vi "init.vi"(8 "error in (no error)":errorcluster, 11 "Relays in":refnum<class "Relays.lvclass">) -> (0 "error out":errorcluster, 3 "Relays out":refnum<class "Relays.lvclass">)   [LabVIEW 2025, in "Relays.lvclass"]
uses:
  Relays.lvclass
  Relays.lvclass/Relays.ctl
  Processor/Processor.lvclass
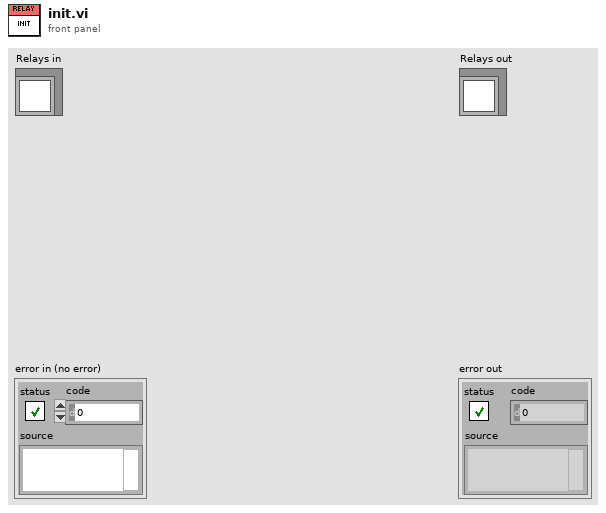
[diagram p1: front panel]
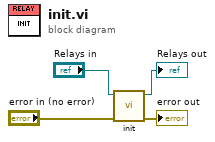
[diagram p0: block diagram]
diagram:
  n1 = call-parent "init.vi"("error in (no error)"="error in (no error)", "Processor in"="Relays in") -> ("error out"=→"error out":errorcluster, "Processor out"=→"Relays out":refnum<class "Relays.lvclass">)  [unwired: 8 in]
